vi "Piano.vi"() -> ()   [LabVIEW 2025]
panel:
  in  "stop":bool
  in  "SI":bool
  in  "LA":bool
  in  "SOL":bool
  in  "FA":bool
  in  "MI":bool
  in  "RE":bool
  in  "DO 2":bool
  in  "DO":bool
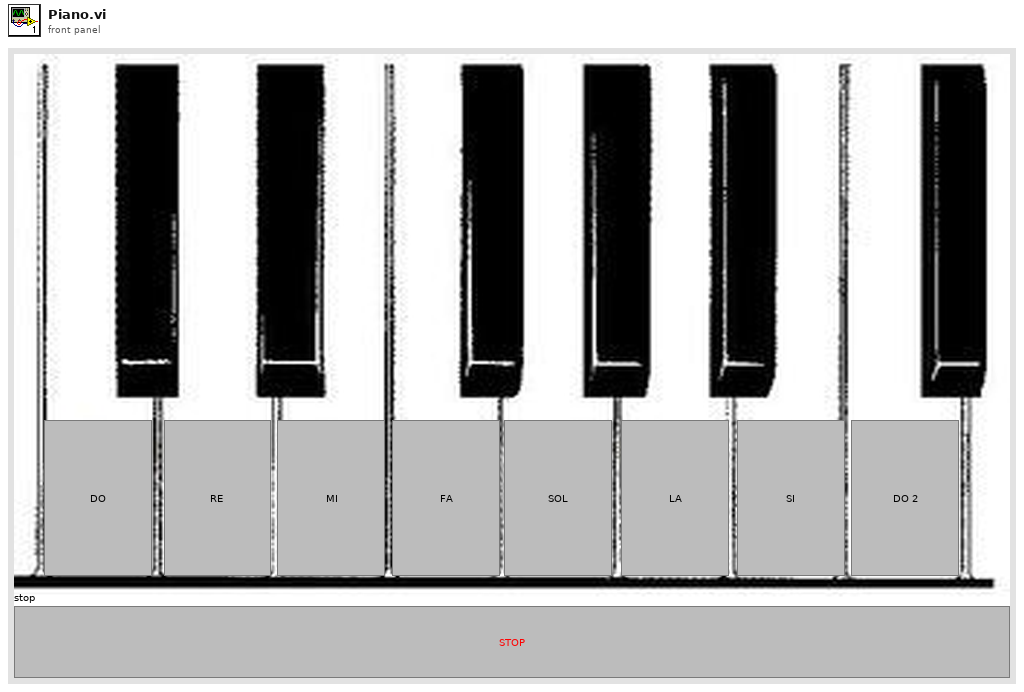
[diagram p1: front panel]
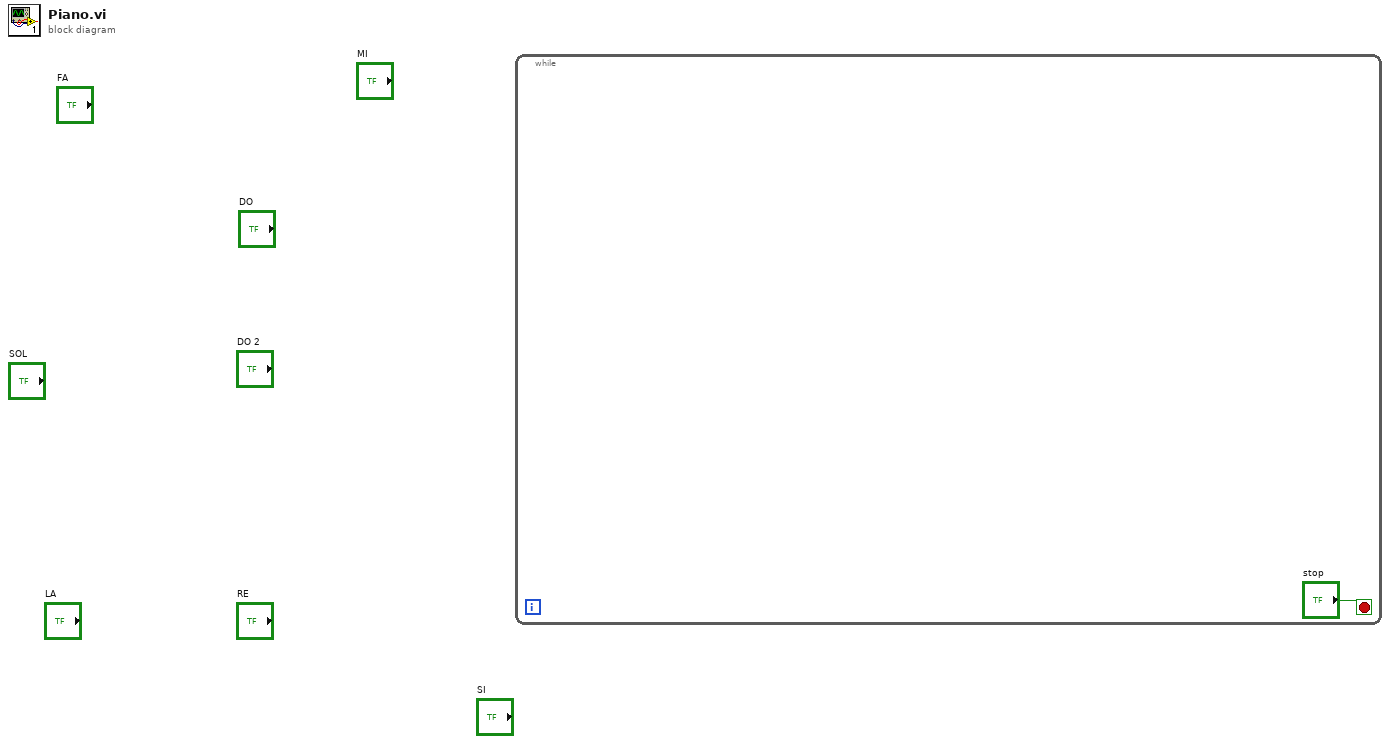
[diagram p0: block diagram]
diagram:
  n1 = while {
    stop <- "stop" stop-if-true
  }
